vi "parse engine statuses.vi"(8 "error in":errorcluster, 11 "message data":string) -> (0 "error out":errorcluster, 3 "engine statuses":T1[](array[typedef]))   [LabVIEW 2013, in "TBD execution service.lvlib"]
doc: "Returns the status of all engines currently loaded by the Engine Service in response to the 'Get Status' command."
uses:
  TBD execution service.lvlib
  engine status data.ctl
  <vilib>/NI/Module Execution Interface/Engine Runtime/Execution States.ctl
  <vilib>/NI/Module Execution Interface/Engine Runtime/Fault.ctl
  <vilib>/NI/Tag Bus Module Framework/runtime/error classification.ctl
  <vilib>/NI/Module Execution Interface/Engine Runtime/Engine Runtime Interface.lvclass
  <vilib>/NI/Tag Bus Module Framework/runtime/TBM module execution interface.lvclass
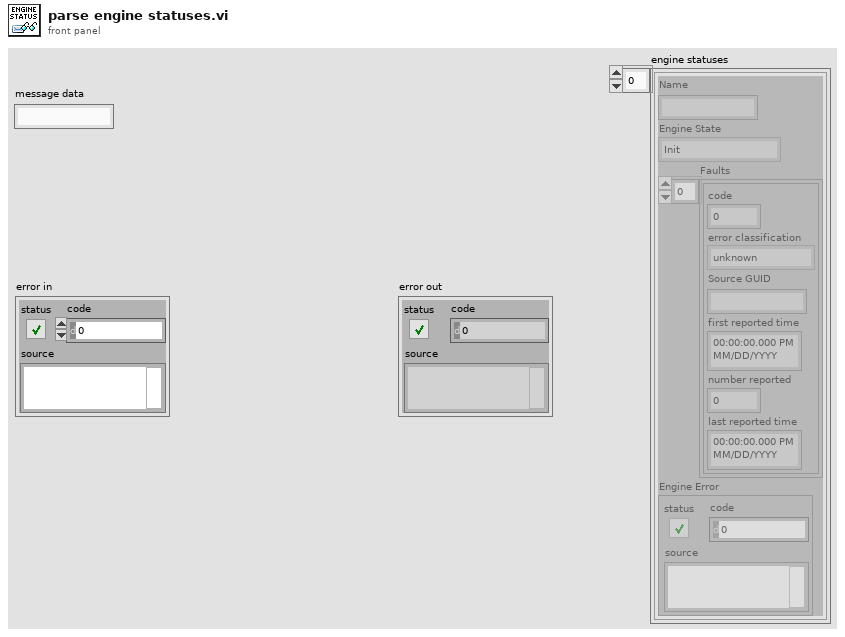
[diagram p1: front panel]
types:
  T1 = typedef "TBD execution service.lvlib/engine status data.ctl" = cluster{"Name":string, "Engine State":T2, "Faults":T3[], "Engine Error":errorcluster}
  T2 = typedef "Engine Runtime Interface.lvclass/Execution States.ctl" = enum16{"Init", "Pre-Operational", "Safe-Operational", "Operational", "Stopped"}
  T3 = typedef "Engine Runtime Interface.lvclass/Fault.ctl" = cluster{"code":i32, "error classification":T4, "Source GUID":string, "first reported time":timestamp, "number reported":u32, "last reported time":timestamp}
  T4 = typedef "TBM module execution interface.lvclass/error classification.ctl" = enum16{"unknown", "none", "trivial", "recoverable", "critical"}
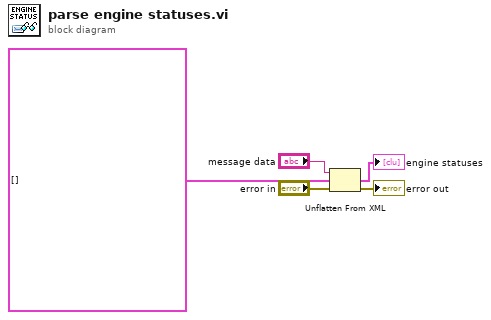
[diagram p0: block diagram]
diagram:
  n1 = Unflatten From XML(xml string="message data", type=T1[] [] ("statuses"), error in (no error)="error in") -> (value=→"engine statuses":T1[], error out=→"error out":errorcluster)
